vi "AI_OneBufferedAI_USB4704 polymorph v1.vi"() -> ()   [LabVIEW 2013]
uses:
  <vilib>/Platform/TimedLoop/XDataNode/timing_clust.ctl
  <vilib>/Platform/TimedLoop/XDataNode/nitl_modes.ctl
  <vilib>/Platform/TimedLoop/XDataNode/wakeup.ctl
  <userlib>/DAQNavi Polymorphic VI/create/DAQNavi Create Channel(AI-Voltage).vi
  <userlib>/DAQNavi Polymorphic VI/configure/timing/DAQNavi Timing(Convert Clock).vi
  <userlib>/DAQNavi Polymorphic VI/read/DAQNavi Read (Analog 1D Wfm NChan NSamp).vi
  <vilib>/platform/TimedLoop/XDataNode/XDataNode.xnode
  <vilib>/Platform/TimedLoop/XDataNode/XDNodeRunTimeDep.lvlib
panel:
  out "Waveform Graph":waveform(dbl)[](graph)
  out "error out":errorcluster
  out "value range":string="+/- 5 V" caption="property value"
  in  "number of samples per channel to read":u32=1000
  in  "samples per channel":i32=1000
  in  "convert clock rate":dbl=1000.0
  out "physical channels":string="DemoDevice,BID#0/ai0:1" caption="property value"
  # "Please modify physical channels and value range in Channel Parameters\nthrough DAQNavi Property Assistant VI  in block diagram."
  # "Channel Parameters"
  # "Timing Parameters"
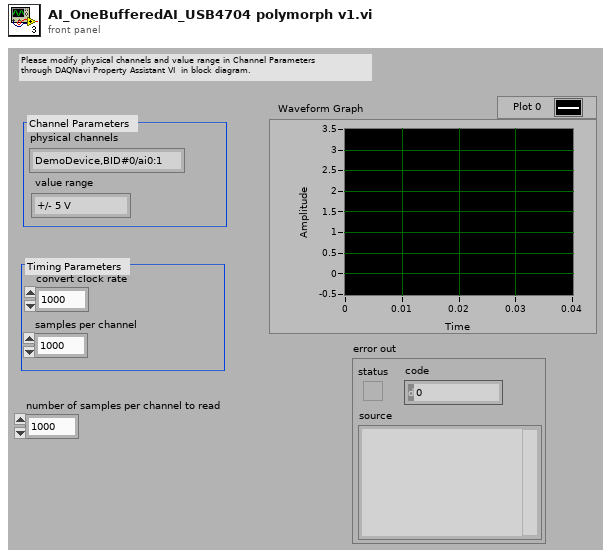
[diagram p1: front panel]
types:
  T1 = typedef "XDNodeRunTimeDep.lvlib/timing_clust.ctl" = cluster{"Expected End [f-1]":u64, "Actual End [f-1]":u64, "Finished Late? [f-1]":bool, "Expected End [i-1]":u64, "Actual End [i-1]":u64, "Finished Late? [i-1]":bool, "Expected Start [i]":u64, "Actual Start [i]":u64, "Expected Start [f]":u64, "Actual Start [f]":u64, "Source Name":string, "Structure Name":string, "Period":i64, "Deadline":i64, "Offset":i64, "Start":i64, "Priority":i32, "Timeout":i32, "Mode":T2, "Wakeup Reason":T3, "Error":errorcluster, "Source Type":string, "Secondary Source Type":string, "Global End Time":u64, "Global Start Time":u64, "Frame Duration":u64, "Iteration Duration":u64, "Assigned CPU":i32, "I/O Scan Engine Mode":u32}
  T2 = typedef "XDNodeRunTimeDep.lvlib/nitl_modes.ctl" = enum32{"No Change", "Process missed periods, maintain original phase", "Discard missed periods, maintain original phase", "Process missed periods, ignore original phase", "Discard missed periods, ignore original phase"}
  T3 = typedef "XDNodeRunTimeDep.lvlib/wakeup.ctl" = enum32{"Normal", "Aborted", "Asynchronous wakeup", "Timing source error", "Timed loop error", "Timeout"}
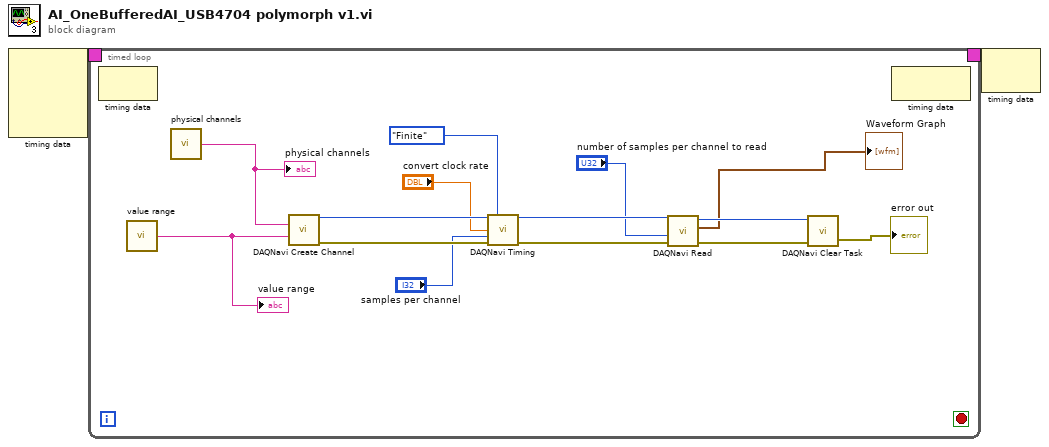
[diagram p0: block diagram]
diagram:
  n1 = node-c288() -> (w2:T1)  [unwired: 4 in]
  n2 = timed-loop {
    timing: w2 -> [_]
    timing-out: [_] -> w1
    stop <- _ stop-if-true
    n3 = node-c288() -> ()  [unwired: 1 in, 1 out]
    n4 = call "value range"() -> ("property value"=w5:string)  [unwired: 1 out]
    "value range" <- w5
    n5 = call "physical channels"() -> ("property value"=w6:string)  [unwired: 1 out]
    "physical channels" <- w6
    n6 = call-poly <userlib>:"DAQNavi Create Channel.vi"("physical channels"=w6, "value range"=w5) -> ("task out"=w14:i32, "error out"=w13:errorcluster)  [unwired: 3 in, 9 out]
    n7 = call-poly <userlib>:"DAQNavi Timing.vi"("task in"=w14, "sample mode"=enum16{"Finite", "Continuous"}."Finite", "rate"="convert clock rate", "samples per channel"="samples per channel", "error in (no error)"=w13) -> ("task out"=w12:i32, "error out"=w11:errorcluster)  [unwired: 1 in, 8 out]
    n8 = call-poly <userlib>:"DAQNavi Read.vi"("error in (no error)"=w11, "number of samples per channel to read"="number of samples per channel to read", "task in"=w12) -> ("error out"=w15:errorcluster, "data"=→"Waveform Graph":waveform(dbl)[], "task out"=w16:i32)  [unwired: 1 in, 5 out]
    n9 = call <userlib>:"DAQNavi Clear Task.vi"("error in (no error)"=w15, "task in"=w16) -> ("error out"=→"error out":errorcluster)  [unwired: 1 out]
    n10 = node-c288() -> ()  [unwired: 1 in, 1 out]
  }
  n11 = node-c288(w1) -> ()  [unwired: 1 out]
